vi "Move absolute.vi"(6 "error in":errorcluster, 7 "New target position (units)":dbl format="%.2f", 8 "Axis in":i32=1, 9 "VISA Handle in":refnum<visa-resource-name>) -> (0 "error out":errorcluster, 2 "Axis out":i32=1, 3 "VISA Handle out":refnum<visa-resource-name>, 4 "TimeoutFlag":bool)   [LabVIEW 2018]
doc: "This VI allows to select a target position. This command is only accepted in READY state. If it is higher or equal to negative software limit and lower or equal to positive software limit, the controller will move the positioner to the selected target position.\nTo avoid any mismatch, the controller when it calculates the new target position will round it to the nearest encoder position."
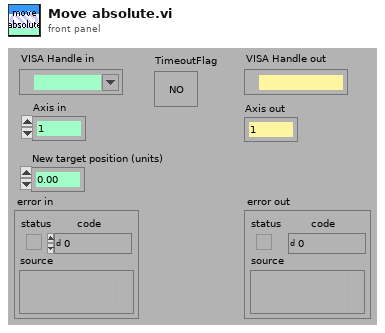
[diagram p1: front panel]
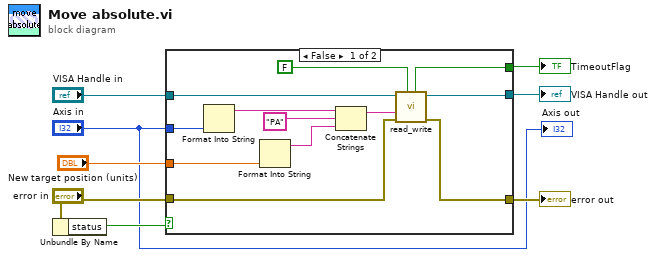
[diagram p0: block diagram]
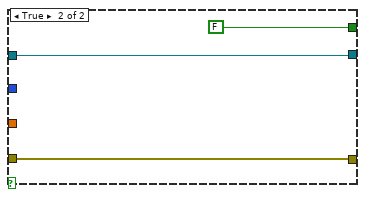
[diagram p2: hidden frame]
diagram:
  n1 = Unbundle By Name("error in") -> ("status"=w6:bool)
  n2 = case shown="False" w6 {
    tunnel: [w16 w23] -> w8
    tunnel: [w15 w22] -> w7
    tunnel: "VISA Handle in" -> [w19 w23]
    tunnel: "error in" -> [w17 w22]
    tunnel: [w14 FALSE ("TimeoutFlag")] -> w3
    tunnel: "Axis in" -> [w9 _]
    tunnel: "New target position (units)" -> [w10 _]
    frame False {
      n3 = Format Into String(w9) -> (resulting string=w12:string)  [unwired: 3 in, 1 out]
      n4 = Format Into String(w10) -> (resulting string=w11:string)  [unwired: 3 in, 1 out]
      n5 = Concatenate Strings(w12, "PA" ("string"), w11) -> (w18:string)
      n6 = call "read_write.vi"("Query?"=FALSE, "error in"=w17, "Command"=w18, "VISA handle in"=w19) -> ("error out"=w15:errorcluster, "VISA handle out"=w16:refnum<visa-resource-name>, "TimeoutFlag"=w14:bool)  [unwired: 2 in, 1 out]
    }
    frame True {
    }
  }
  "VISA Handle out" <- w8
  "error out" <- w7
  "TimeoutFlag" <- w3
  "Axis out" <- "Axis in"
